vi "Do.vi"(8 "error in (no error)":errorcluster, 10 "Actor in":refnum<class "Actor.lvclass">, 11 "Initialize Force Task Msg in":refnum<class "Initialize Force Task Msg.lvclass">) -> (0 "error out":errorcluster, 2 "Actor out":refnum<class "Actor.lvclass">)   [LabVIEW 2020, in "NI Force Task.lvlib" / "Initialize Force Task Msg.lvclass"]
doc: "(<B>Filename</B>: Actor Framework.lvlib:Message.lvclass:Do.vi)\n\nDefines what a message does when it is received by an actor. Generally, a message instructs an actor to invoke one of its methods. By default, this method does nothing. A child class must override it to define behavior. Create a child class by using the Actor Framework Message Maker dialog box."
uses:
  Initialize Force Task Msg.lvclass
  <vilib>/ActorFramework/Actor/Actor.lvclass
  NI Force Task/NI Force Task.lvclass
  C:/Program Files/National Instruments/LabVIEW 2020/vi.lib/ActorFramework/Actor/Actor.lvclass
  Initialize Force Task Msg.lvclass/Initialize Force Task Msg.ctl
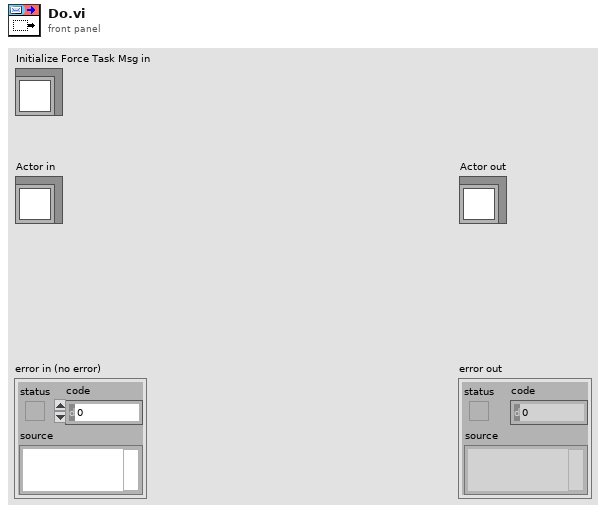
[diagram p1: front panel]
types:
  T1 = cluster{"Force Transducer: Left":tag, "Force Transducer: Right ":tag, "EMG: Left":tag, "EMG: Right":tag, "Potentiometer: Left":tag, "Potentiometer: Right":tag}
  T2 = typedef "Task info df.ctl" = cluster{"Number of Trials":u8, "Sampling Rate (Hz)":u16, "Trial Duration (s)":u8, "Adjusted MVC (N)":dbl, "R Phase":i32, "L Phase":i32, "L Pattern":u8, "R Pattern":u8, "Time Between Trials (s)":u8, "Lissajous Speed":u16}
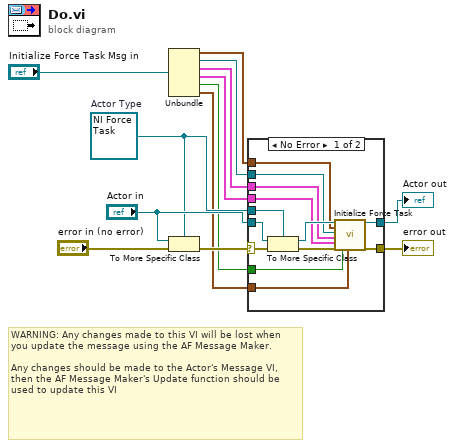
[diagram p0: block diagram]
diagram:
  w8 = refnum<class "NI Force Task.lvclass"> refnum  # Actor Type
  # "WARNING: Any changes made to this VI will be lost when you update the message using the AF Message Maker.\n\nAny changes should be made to the Actor's Message VI, then the AF Message Maker's Update function should be used to update this VI"
  n1 = Unbundle("Initialize Force Task Msg in") -> (w7:cluster{"Left":dbl, "Right":dbl}, w6:refnum<k34>, w5:cluster{"Collect EMG?":bool, "EMG Rate":u16}, w4:T1, w3:bool, w2:T2)
  n2 = To More Specific Class(target class=w8, reference="Actor in", error in="error in (no error)") -> (error out=w12:errorcluster)  [unwired: 1 out]
  n3 = case shown="No Error" w12 {
    selector: w12 -> [w26 w28]
    tunnel: [w21 w28] -> w11
    tunnel: [w20 w27] -> w10
    tunnel: "Actor in" -> [w25 w27]
    tunnel: w8 -> [w24 _]
    tunnel: w7 -> [w19 _]
    tunnel: w6 -> [w18 _]
    tunnel: w5 -> [w17 _]
    tunnel: w4 -> [w16 _]
    tunnel: w3 -> [w15 _]
    tunnel: w2 -> [w14 _]
    frame No Error {
      n4 = To More Specific Class ("Actor Cast")(target class=w24, reference=w25, error in=w26) -> (specific class reference=w23:refnum<class "NI Force Task.lvclass">, error out=w22:errorcluster)
      n5 = call "Initialize Force Task.vi"("NI Force Task in"=w23, "Force Calibration Cluster"=w19, "TDMS File"=w18, "EMG info"=w17, "DAQ  Channels In"=w16, "error in (no error)"=w22, "Scanning?"=w15, "Task Info In"=w14) -> ("NI Force Task out"=w20:refnum<class "NI Force Task.lvclass">, "error out"=w21:errorcluster)  [unwired: 10 in]
    }
    frame Error {
    }
  }
  "error out" <- w11
  "Actor out" <- w10
